vi "afmmode - testbench.vi"() -> ()   [LabVIEW 2019]
uses:
  <userlib>/HapticSTM/HapticSTM.lvlib
panel:
  out "force":dbl
  out "Z Write (m) 2":dbl
  in  "Z Write?":bool
  in  "Save":bool
  in  "# Sample Points":i32=4096
  out "Signal value":sgl format="%#_6p"
  out "Z Write (m)":dbl
  in  "Signal index (0-127)":i8
  in  "Upper Limit (mm)":dbl=50.0
  in  "Lower Limit (mm)":dbl=-40.0
  in  "Upper Limit (nm)":dbl=1.0
  in  "Lower Limit (nm)":dbl
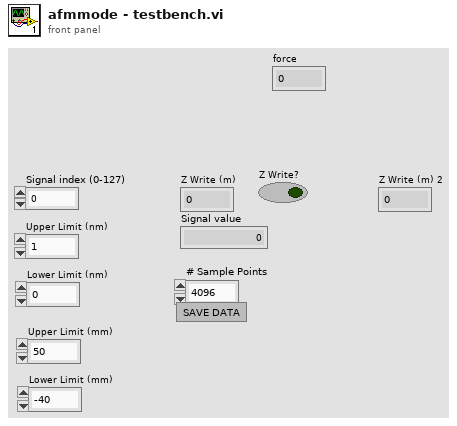
[diagram p1: front panel]
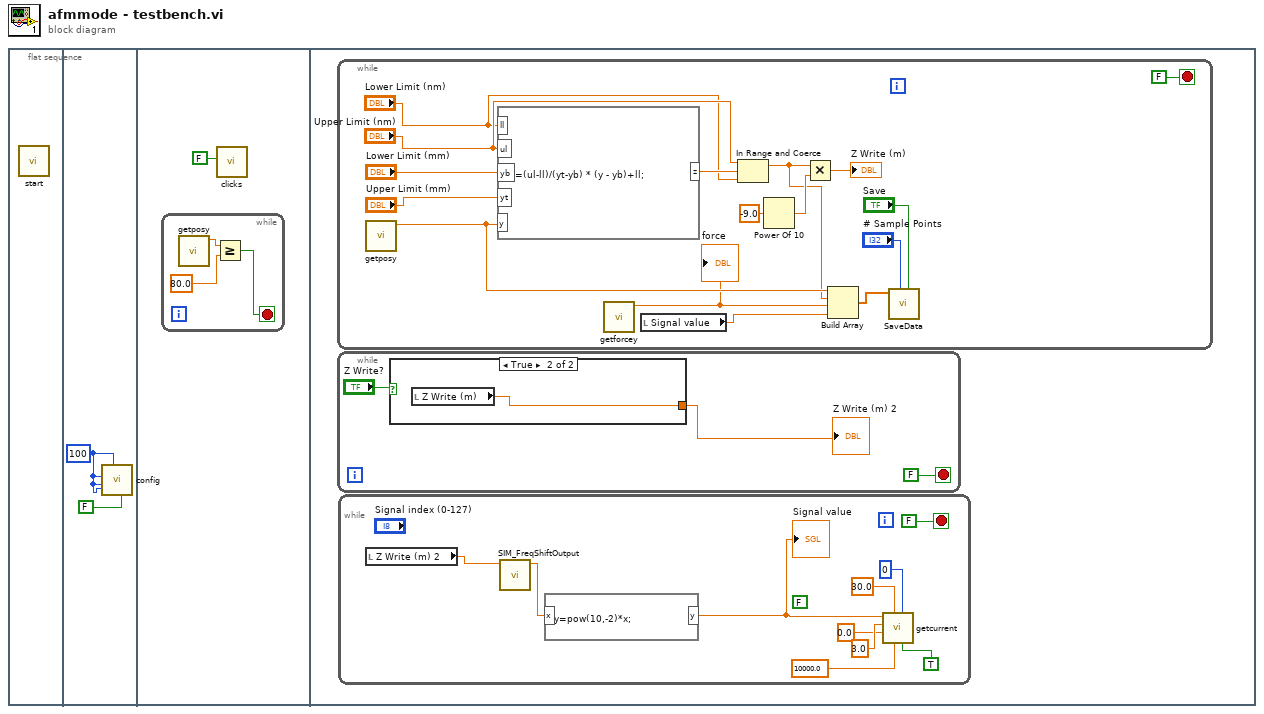
[diagram p0: block diagram]
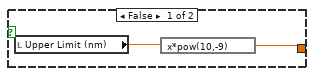
[diagram p2: hidden frame]
diagram:
  n1 = flat-sequence {
    frame #0 {
      n2 = call <userlib>:"start.vi"() -> ()  [unwired: 11 in, 1 out]
    }
    frame #1 {
      w1 = 100 ("sizeofimgx")
      n3 = call <userlib>:"config.vi"("feedback"=FALSE, "sizeofimgz"=w1, "sizeofimgx"=w1, "scopez"=w1, "scopex"=w1) -> ()  [unwired: 7 in]
    }
    frame #2 {
      n4 = while {
        stop <- w4 stop-if-true
        n5 = call <userlib>:"getposy.vi"() -> ("function return"=w6:dbl)  [unwired: 11 in]
        n6 = Greater Or Equal?(x=w6, y=80.0) -> (x >= y?=w4:bool)
      }
      n7 = call <userlib>:"clicks.vi"("planing"=FALSE) -> ()  [unwired: 10 in, 1 out]
    }
    frame #3 {
      n8 = while {
        stop <- FALSE stop-if-true
        n9 = call <userlib>:"getposy.vi"() -> ("function return"=w29:dbl)  [unwired: 11 in]
        n10 = formula code="z =(ul-ll)/(yt-yb) * (y - yb)+ll;"("ll"="Lower Limit (nm)", "ul"="Upper Limit (nm)", "yb"="Lower Limit (mm)", "yt"="Upper Limit (mm)", "y"=w29) -> ("z"=w33:dbl)
        n11 = call <userlib>:"getforcey.vi"() -> ("function return"=w27:dbl)  [unwired: 11 in]
        "force" <- w27
        n12 = local read "Signal value"() -> (w24:sgl)
        n13 = In Range and Coerce(upper limit="Upper Limit (nm)", x=w33, lower limit="Lower Limit (nm)") -> (coerced(x)=w28:dbl)  [unwired: 1 out]
        n14 = Power Of 10(x=-9.0) -> (10^x=w34:dbl)
        n15 = Multiply(x=w28, y=w34) -> (x*y=→"Z Write (m)":dbl)
        n16 = Build Array(w29, w28, w27, w24) -> (w23:dbl[])
        n17 = call "SaveData.vi"("Save"="Save", "# Sample Points"="# Sample Points", "Data"=w23) -> ()  [unwired: 9 in]
      }
      n18 = while {
        stop <- FALSE stop-if-true
        n19 = case shown="True" "Z Write?" {
          tunnel: [w10 w12] -> w9
          frame False {
            n20 = local read "Upper Limit (nm)"() -> (w11:dbl)
            n21 = expression code="x*pow(10,-9)"(w11) -> (w10:dbl)
          }
          frame True {
            n22 = local read "Z Write (m)"() -> (w12:dbl)
          }
        }
        "Z Write (m) 2" <- w9
      }
      n23 = while {
        stop <- FALSE stop-if-true
        (unwired) FALSE ("feedback")
        n24 = local read "Z Write (m) 2"() -> (w14:dbl)
        n25 = call "SIM_FreqShiftOutput.vi"("zin (m)"=w14) -> ("Current Out (pA)"=w19:dbl)  [unwired: 10 in]
        n26 = formula code="y=pow(10,-2)*x;"("x"=w19) -> ("y"=w13:dbl)
        "Signal value" <- w13
        n27 = call <userlib>:"getcurrent.vi"("afmmode"=TRUE, "forcemode"=0, "maxcurrentin"=10000.0, "setpoint"=30.0, "minforcey"=0.0, "maxforcey"=3.0, "currentin"=w13) -> ()  [unwired: 5 in]
      }
    }
  }
